vi "Retention Test.vi"(5 "Current address":i32, 6 "WL voltage (V)":dbl, 7 "target outfile":path, 8 "error in (no error)":errorcluster, 9 "final resistance (ohm)":dbl, 10 "SL voltage (V)":dbl, 11 "IVI Refnum in":refnum<k15>) -> (0 "error out":errorcluster, 3 "IVI Refnum out":refnum<k15>)   [LabVIEW 2018]
uses:
  <vilib>/Utility/file.llb/Write Delimited Spreadsheet (DBL).vi
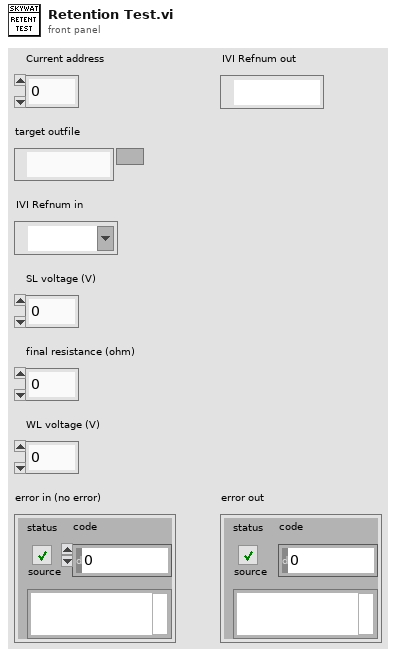
[diagram p1: front panel]
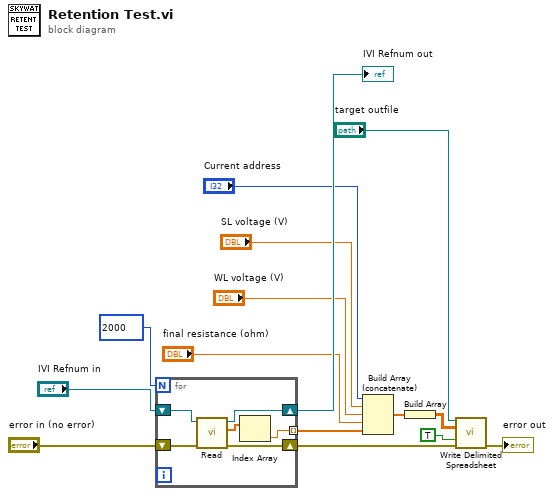
[diagram p0: block diagram]
diagram:
  n1 = for {
    N: 2000 -> [_]
    tunnel: [w19] -> w6 mode=indexing
    shift-right: [w18] -> w7
    shift-left: "error in (no error)" -> [w16]
    shift-right: [w17] -> w15
    shift-left: "IVI Refnum in" -> [w20]
    n2 = call "Read.vi"("error in (no error)"=w16, "instrument handle"=w20) -> ("error out"=w18:errorcluster, "resistances (ohm)"=w21:dbl[], "instrument handle out"=w17:refnum<k15>)  [unwired: 6 in, 1 out]
    n3 = Index Array(array=w21) -> (element=w19:dbl)  [unwired: 1 in]
  }
  "IVI Refnum out" <- w15
  n4 = Build Array (concatenate)("Current address", "SL voltage (V)", "WL voltage (V)", "final resistance (ohm)", w6) -> (w1:dbl[])
  n5 = Build Array(w1) -> (w2:dbl[][])
  n6 = call-poly <vilib>:"Write Delimited Spreadsheet.vi"("file path (dialog if empty)"="target outfile", "2D data"=w2, "append to file? (new file:F)"=TRUE, "error in (no error)"=w7) -> ("error out"=→"error out":errorcluster)  [unwired: 10 in, 1 out]
